vi "RGB_to_V.vi"(1 "BLUE":u16, 2 "GREEN":u16, 3 "RED":u16) -> (0 "无符号16位整型":u16)   [LabVIEW 2018]
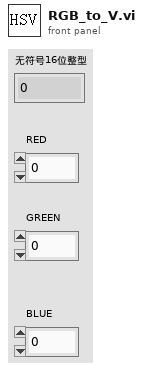
[diagram p1: front panel]
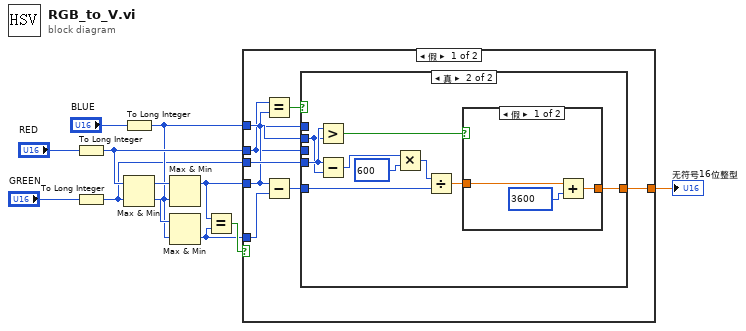
[diagram p0: block diagram]
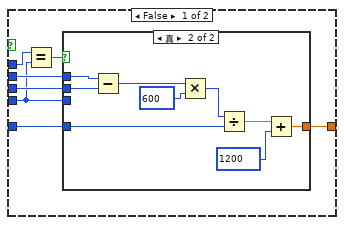
[diagram p2: hidden frame]
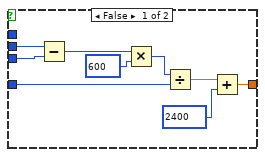
[diagram p3: hidden frame]
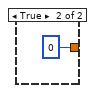
[diagram p5: hidden frame]
diagram:
  n1 = To Long Integer(number="RED") -> (32bit integer=w6:i32)
  n2 = To Long Integer(number="GREEN") -> (32bit integer=w2:i32)
  n3 = To Long Integer(number="BLUE") -> (32bit integer=w4:i32)
  n4 = Max & Min(x=w6, y=w2) -> (max(x,y)=w12:i32, min(x,y)=w11:i32)
  n5 = Max & Min(x=w12, y=w4) -> (max(x,y)=w9:i32)  [unwired: 1 out]
  n6 = Max & Min(x=w11, y=w4) -> (min(x,y)=w8:i32)  [unwired: 1 out]
  n7 = Equal?(x=w9, y=w8) -> (x = y?=w10:bool)
  n8 = case shown="假" w10 {
    tunnel: [w16 u16 0] -> w7
    tunnel: w6 -> [w13 _]
    tunnel: w2 -> [w19 _]
    tunnel: w4 -> [w18 _]
    tunnel: w9 -> [w15 _]
    tunnel: w8 -> [w17 _]
    frame False {
      n9 = Equal?(x=w13, y=w15) -> (x = y?=w20:bool)
      n10 = Subtract(x=w15, y=w17) -> (x-y=w14:i32)
      n11 = case shown="真" w20 {
        tunnel: w19 -> [w21 w48]
        tunnel: w18 -> [w25 w47]
        tunnel: [w22 w52] -> w16
        tunnel: w15 -> [w27 _]
        tunnel: w14 -> [w23 w51]
        tunnel: w13 -> [w24 _]
        frame False {
          n12 = Equal?(x=w27, y=w21) -> (x = y?=w26:bool)
          n13 = case shown="真" w26 {
            tunnel: w25 -> [_ w45]
            tunnel: w24 -> [w36 w44]
            tunnel: w23 -> [w32 w41]
            tunnel: [w28 w37] -> w22
            tunnel: w21 -> [w35 _]
            frame False {
              n14 = Subtract(x=w36, y=w35) -> (x-y=w34:i32)
              n15 = Multiply(x=w34, y=600) -> (x*y=w31:i32)
              n16 = Divide(x=w31, y=w32) -> (x/y=w29:dbl)
              n17 = Add(x=w29, y=2400) -> (x+y=w28:dbl)
            }
            frame True {
              n18 = Subtract(x=w45, y=w44) -> (x-y=w42:i32)
              n19 = Multiply(x=w42, y=600) -> (x*y=w40:i32)
              n20 = Divide(x=w40, y=w41) -> (x/y=w38:dbl)
              n21 = Add(x=w38, y=1200) -> (x+y=w37:dbl)
            }
          }
        }
        frame True {
          n22 = Greater?(x=w48, y=w47) -> (0:w46:bool)
          n23 = Subtract(x=w48, y=w47) -> (x-y=w53:i32)
          n24 = Multiply(x=w53, y=600) -> (x*y=w50:i32)
          n25 = Divide(x=w50, y=w51) -> (x/y=w49:dbl)
          n26 = case shown="假" w46 {
            tunnel: [w55 w58] -> w52
            tunnel: w49 -> [w56 w58]
            frame False {
              n27 = Add(x=w56, y=3600) -> (x+y=w55:dbl)
            }
            frame True {
            }
          }
        }
      }
    }
    frame True {
    }
  }
  "无符号16位整型" <- w7
